vi "DBReadStringAsNumber.vi"(10 "Default Value":dbl, 11 "DBControlName":string="String") -> (3 "Value":dbl)   [LabVIEW 2016]
uses:
  <vilib>/Rock Robotics/Network Tables/NT Read String.vi
  <vilib>/Rock Robotics/Network Tables/NT Write String.vi
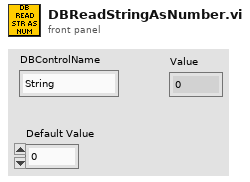
[diagram p1: front panel]
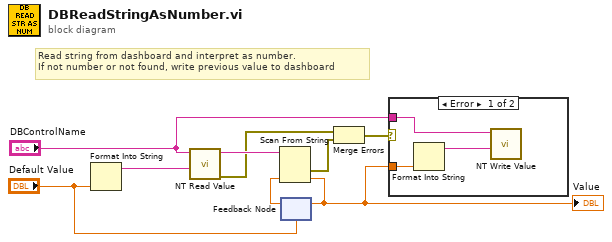
[diagram p0: block diagram]
diagram:
  # "Read string from dashboard and interpret as number.\nIf not number or not found, write previous value to dashboard"
  n1 = Format Into String("Default Value") -> (resulting string=w9:string)  [unwired: 3 in, 1 out]
  n2 = call-poly <vilib>:"NT Read Value.vi"("Default Value"=w9, "Name"="DBControlName") -> ("error out"=w5:errorcluster, "String"=w8:string)  [unwired: 8 in]
  n3 = feedback #1("Default Value") -> (w7:dbl)
  n4 = Scan From String(input string=w8, default 1=w7) -> (error out=w4:errorcluster, output 1=w3:dbl)  [unwired: 3 in, 2 out]
  "Value" <- w3
  n5 = feedback-in #1(w3) -> ()
  n6 = Merge Errors(w5, w4) -> (w1:errorcluster)
  n7 = case shown="Error" w1 {
    tunnel: w3 -> [w12 _]
    tunnel: "DBControlName" -> [w10 _]
    frame Error {
      n8 = Format Into String(w12) -> (resulting string=w11:string)  [unwired: 3 in, 1 out]
      n9 = call-poly <vilib>:"NT Write Value.vi"("String"=w11, "Name"=w10) -> ()  [unwired: 9 in, 1 out]
    }
    frame No Error {
    }
  }
